vi "VIC_IRQ.vi"(7 "oper":T1, 10 "IRQ flag idx":u8 format="%.0b", 11 "mask value":u8 format="%.0b") -> (1 "IRQ.active":bool, 2 "IRQ.reg":u8 format="%08b", 3 "IRQ.mask":u8 format="%08b")   [LabVIEW 2018]
uses:
  VIC_IRQ_oper.ctl
  VIC_glb.vi
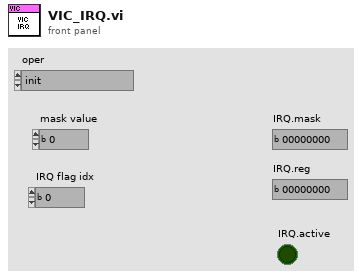
[diagram p1: front panel]
types:
  T1 = typedef "VIC_IRQ_oper.ctl" = enum16{"init", "set mask", "set flag", "check active", "read reg", "reset flag"}
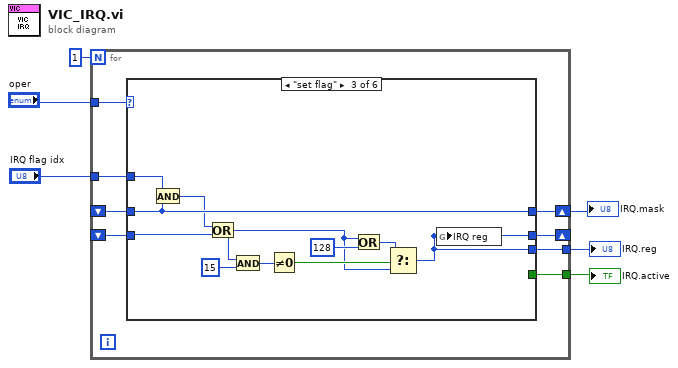
[diagram p0: block diagram]
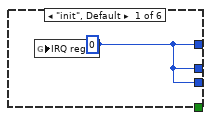
[diagram p2: hidden frame]
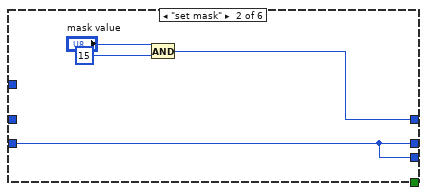
[diagram p3: hidden frame]
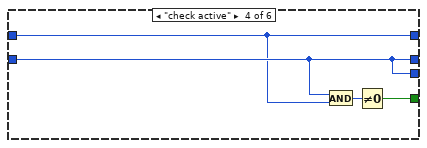
[diagram p4: hidden frame]
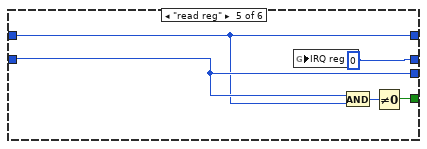
[diagram p5: hidden frame]
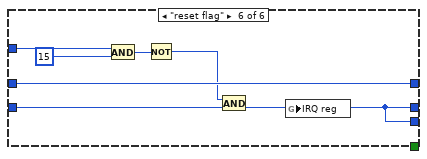
[diagram p6: hidden frame]
diagram:
  n1 = for {
    N: 1 -> [_]
    shift-right: [w13] -> w4
    shift-left: _ -> [w12]
    tunnel: "oper" -> [w14]
    shift-right: [w8] -> _
    shift-left: _ -> [w11]
    tunnel: "IRQ flag idx" -> [w10]
    tunnel: [w9] -> w2
    tunnel: [w7] -> w1
    n2 = case shown="\"set flag\"" w14 {
      tunnel: [w15 w16 w22 w31 w35 w46] -> w13
      tunnel: w12 -> [_ _ w22 w31 w35 w46]
      tunnel: w11 -> [_ w18 w30 w32 w37 w41]
      tunnel: [w15 w18 w23 w32 w36 w40] -> w8
      tunnel: w10 -> [_ _ w20 _ _ w44]
      tunnel: [_ _ _ w34 w38 _] -> w9
      tunnel: [w15 w18 w23 w32 w37 w40] -> w7
      frame "init", Default {
        w15 = u8 0 ("mask")
        n3 = global write "VIC_glb.vi" "IRQ reg"(w15) -> ()
      }
      frame "set mask" {
        n4 = And(x="mask value", y=u8 15) -> (x .and. y?=w16:u8)
      }
      frame "set flag" {
        n5 = And(x=w20, y=w22) -> (x .and. y?=w21:u8)
        n6 = Or(x=w21, y=w30) -> (x .or. y?=w24:u8)
        n7 = And(x=w24, y=u8 15) -> (x .and. y?=w28:u8)
        n8 = Not Equal To 0?(x=w28) -> (x != 0?=w26:bool)
        n9 = Or(x=w24, y=u8 128) -> (x .or. y?=w25:u8)
        n10 = Select(t=w25, s=w26, f=w24) -> (s? t:f=w23:u8)
        n11 = global write "VIC_glb.vi" "IRQ reg"(w23) -> ()
      }
      frame "check active" {
        n12 = And(x=w32, y=w31) -> (x .and. y?=w33:u8)
        n13 = Not Equal To 0?(x=w33) -> (x != 0?=w34:bool)
      }
      frame "read reg" {
        w36 = u8 0 ("mask")
        n14 = global write "VIC_glb.vi" "IRQ reg"(w36) -> ()
        n15 = And(x=w37, y=w35) -> (x .and. y?=w39:u8)
        n16 = Not Equal To 0?(x=w39) -> (x != 0?=w38:bool)
      }
      frame "reset flag" {
        n17 = And(x=w44, y=u8 15) -> (x .and. y?=w43:u8)
        n18 = Not(x=w43) -> (.not. x?=w42:u8)
        n19 = And(x=w42, y=w41) -> (x .and. y?=w40:u8)
        n20 = global write "VIC_glb.vi" "IRQ reg"(w40) -> ()
      }
    }
  }
  "IRQ.mask" <- w4
  "IRQ.reg" <- w1
  "IRQ.active" <- w2
